vi "measure_voltage.vi"(0 "VISA resource name":refnum<visa-resource-name>) -> ()   [LabVIEW 2020]
uses:
  controls/SCPI_enum.ctl
panel:
  out "Waveform Chart 2":dbl(graph)
  out "Waveform Chart":dbl(graph)
  out "Array":dbl[][](array[numeric])
  out "error out":errorcluster
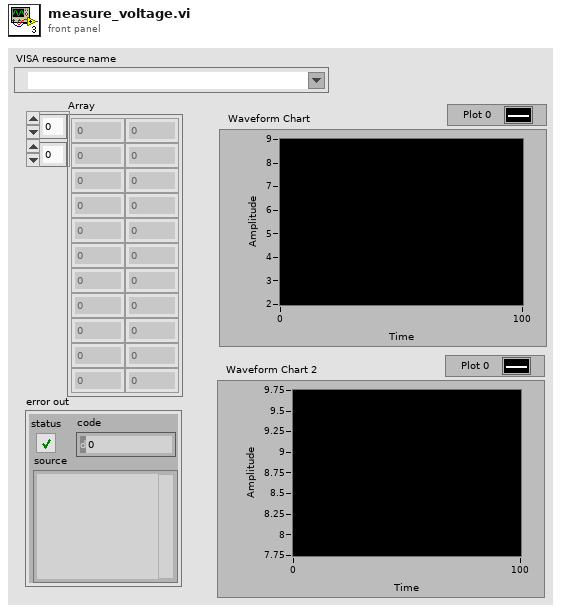
[diagram p1: front panel]
types:
  T1 = typedef "SCPI_enum.ctl" = u16
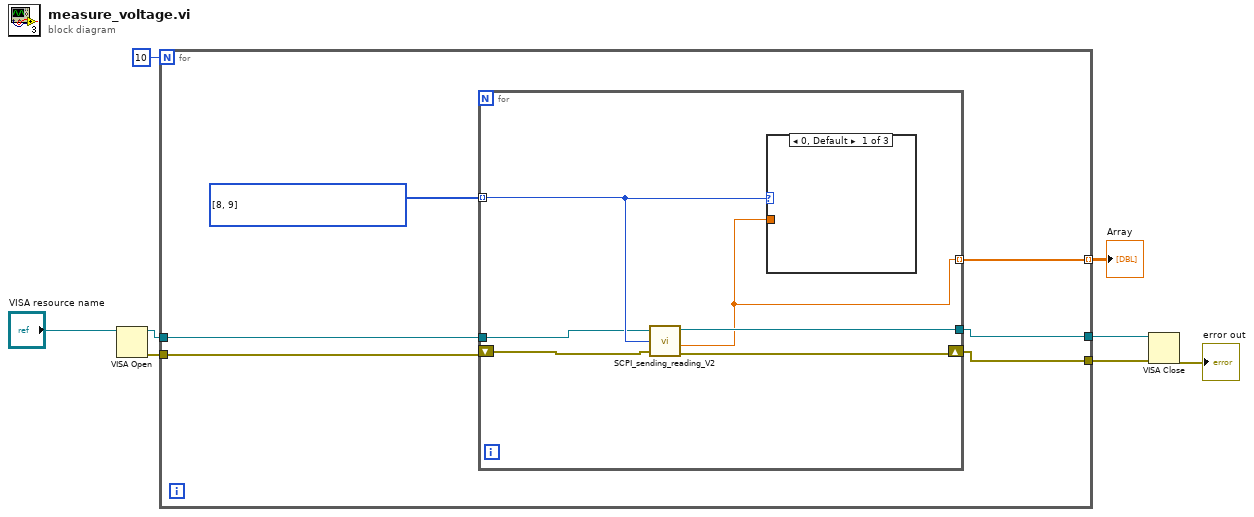
[diagram p0: block diagram]
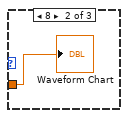
[diagram p2: hidden frame]
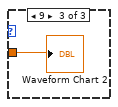
[diagram p3: hidden frame]
diagram:
  n1 = VISA Open(VISA resource name="VISA resource name") -> (VISA resource name=w2:refnum<visa-resource-name>, error out=w1:errorcluster)  [unwired: 4 in]
  n2 = for {
    N: 10 -> [_]
    tunnel: [w13] -> w7 mode=indexing
    tunnel: [w12] -> w5
    tunnel: [w11] -> w4
    tunnel: w2 -> [w10]
    tunnel: w1 -> [w9]
    w14 = T1[] [8, 9] items=["*IDN?", "*SAV 1", "*RCL 1", "INSTTrument CH1", "INSTTrument CH2", "INSTrument?", "MEASure:CURRent? CH1", "MEASure:CURRent? CH2", "MEASure:VOLTage? CH1", "MEASure:VOLTage? CH2", "MEASure:POWEr? CH1", "MEASure:POWEr? CH2", "CH1:CURRent?", "CH2:CURRent?", "CH1:VOLTage? ", "CH2:VOLTage? ", "OUTPut CH1,ON", "OUTPut CH1,OFF", "OUTPut CH2,ON", "OUTPut CH2,OFF", "OUTPut CH3,ON", "OUTPut CH3,OFF", "OUTPut:TRACK 0", "OUTPut:TRACK 1", "OUTPut:TRACK 2", "OUTPut:WAVE CH1,ON", "OUTPut:WAVE CH1,OFF", "OUTPut:WAVE CH2,ON", "OUTPut:WAVE CH2,OFF", "CH1:VOLTage", "CH2:VOLTage", "CH1:CURRent", "CH2:CURRent"]
    n3 = for {
      tunnel: w14 -> [w17] mode=indexing
      tunnel: [w19] -> w11
      shift-right: [w18] -> w12
      shift-left: w9 -> [w20]
      tunnel: [w16] -> w13 mode=indexing
      tunnel: w10 -> [w15]
      n4 = call "SCPI_sending_reading_V2.vi"("VISA"=w15, "SCIPI"=w17, "error in (no error)"=w20) -> ("VISA resource name out"=w19:refnum<visa-resource-name>, "read numeric value"=w16:dbl, "error out"=w18:errorcluster)  [unwired: 1 out]
      n5 = case shown="0, Default" w17 {
        tunnel: w16 -> [_ w21 w22]
        frame 0, Default {
        }
        frame 8 {
          "Waveform Chart" <- w21
        }
        frame 9 {
          "Waveform Chart 2" <- w22
        }
      }
    }
  }
  "Array" <- w7
  n6 = VISA Close(VISA resource name=w4, error in (no error)=w5) -> (error out=→"error out":errorcluster)
